vi "CreateDiagrams.vi"(6 "error in":errorcluster, 9 "WhileLoop in":refnum<class "WhileLoop.lvclass">) -> (0 "error out":errorcluster, 3 "WhileLoop out":refnum<class "WhileLoop.lvclass">, 4 "create_diagrams":string)   [LabVIEW 2014, in "Raspberry Pi Compatible Compiler for LabVIEW.lvlib" / "WhileLoop.lvclass"]
uses:
  WhileLoop.lvclass
  Python/Parsing/ClassTypeTD.ctl
  Structure/Structure.lvclass/Structure.ctl
  Diagram/Diagram.lvclass
  Structure/Structure.lvclass
  Python/Parsing/Python Functions.lvlib
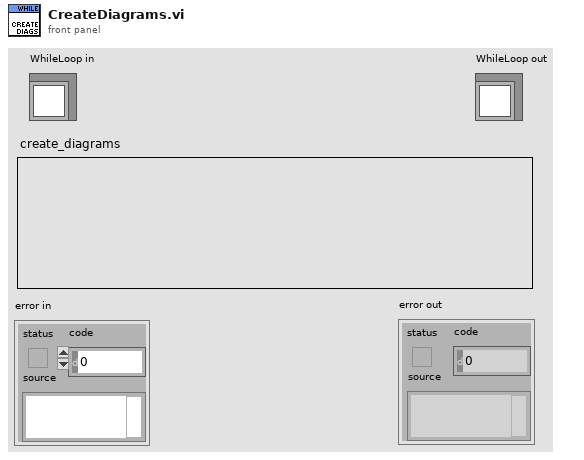
[diagram p1: front panel]
types:
  T1 = typedef "Raspberry Pi Compatible Compiler for LabVIEW.lvlib/Python Functions.lvlib/ClassTypeTD.ctl" = enum16{"class", "function"}
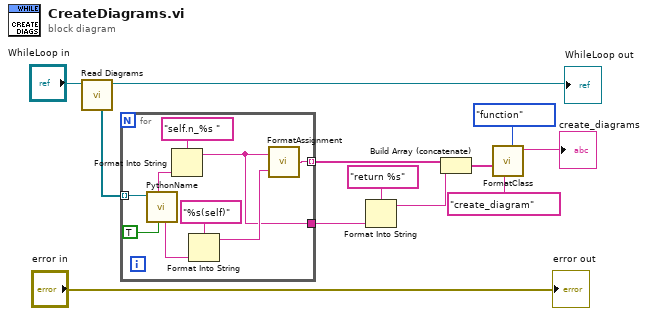
[diagram p0: block diagram]
diagram:
  n1 = call "Read Diagrams.vi"("Structure in"="WhileLoop in") -> ("Structure out"=→"WhileLoop out":refnum<class "WhileLoop.lvclass">, "Diagrams"=w12:refnum<class "Diagram.lvclass">[])  [unwired: 7 in]
  n2 = for {
    tunnel: w12 -> [w21] mode=indexing
    tunnel: [w17] -> w5 mode=indexing
    tunnel: [w13] -> w3
    n3 = call-dynamic "PythonName.vi"("add self"=TRUE, "Diagram in"=w21) -> ("name"=w16:string, "UID"=w18:string)  [unwired: 6 in, 2 out]
    n4 = Format Into String(format string="self.n_%s ", w18) -> (resulting string=w13:string)  [unwired: 2 in, 1 out]
    n5 = Format Into String(format string="%s(self)", w16) -> (resulting string=w14:string)  [unwired: 2 in, 1 out]
    n6 = call "FormatAssignment.vi"("value"=w14, "name"=w13) -> ("python assignment"=w17:string)
  }
  n7 = Format Into String(format string="return %s", w3) -> (resulting string=w2:string)  [unwired: 2 in, 1 out]
  n8 = Build Array (concatenate)(w5, w2) -> (w4:string[])
  n9 = call "FormatClass.vi"("type"=ClassTypeTD."function", "name"="create_diagram", "body"=w4) -> ("python"=→"create_diagrams":string)  [unwired: 8 in]
  "error out" <- "error in"
